vi "3D_Traverse_move_manual.vi"() -> ()   [LabVIEW 2020]
uses:
  Controls/Tunnel_Coordinates.ctl
  Trav_mode.ctl
  Controls/User_Specific_mode.ctl
  Globals/Constants_global.vi
panel:
  out "Current Traverse":string
  in  "Work in Tunnel Coordinates":T1
  in  "Traverse":u16(ring) items=["A_Tunnel", "A_Tunnel_Turntable", "Aero_Enclosure", "Aero_Pitch", "Aero_Sting", "Aero_ThroughWall", "Aero_Tunnel", "Angle_Calibrator", "B_Tunnel", "D_Tunnel", "dummy", "Dummy_Traverse", "EnFlo_Stack", "EnFlo_Trav1", "EnFlo_Trav3", "EnFlo_Trav4", "EnFlo_Tunnel", "EnFlo_Turntable", "F1_Wing_Angle", "Fast_Trav", "Fruit_Rig", "Laser_Disp_Scanner", "Laser_Meas_Traverse", "None", "Pitch_Traverse", "Pitch_Yaw", "PIV_Traverse", "Pressure_Port_1", "Pressure_Port_2", "Scanning Valve", "Soil_Rig", "Tank", "Trav_test"]
  in  "stop":bool
  in  "Increment":dbl=10.0
  in  "Z-":bool
  in  "Z+":bool
  in  "Y+":bool
  in  "Y-":bool
  in  "X+":bool
  in  "X-":bool
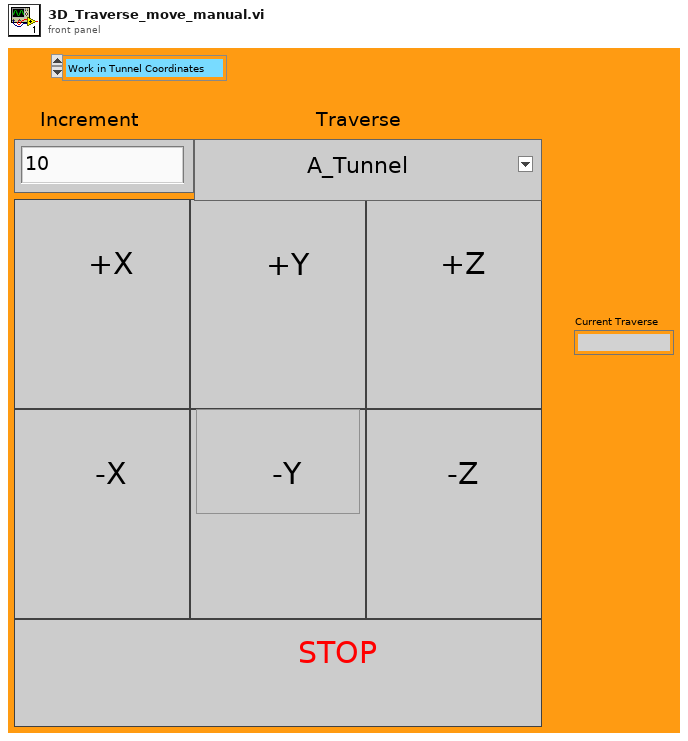
[diagram p1: front panel]
types:
  T1 = typedef "Tunnel_Coordinates.ctl" = enum16{"Work in Tunnel Coordinates", "Work in Model Coordinates"}
  T2 = typedef "User_Specific_mode.ctl" = enum16{"Check VI only", "Run VI"}
  T3 = typedef "Trav_mode.ctl" = enum16{"Move traverse", "Read traverse position", "Teach Position"}
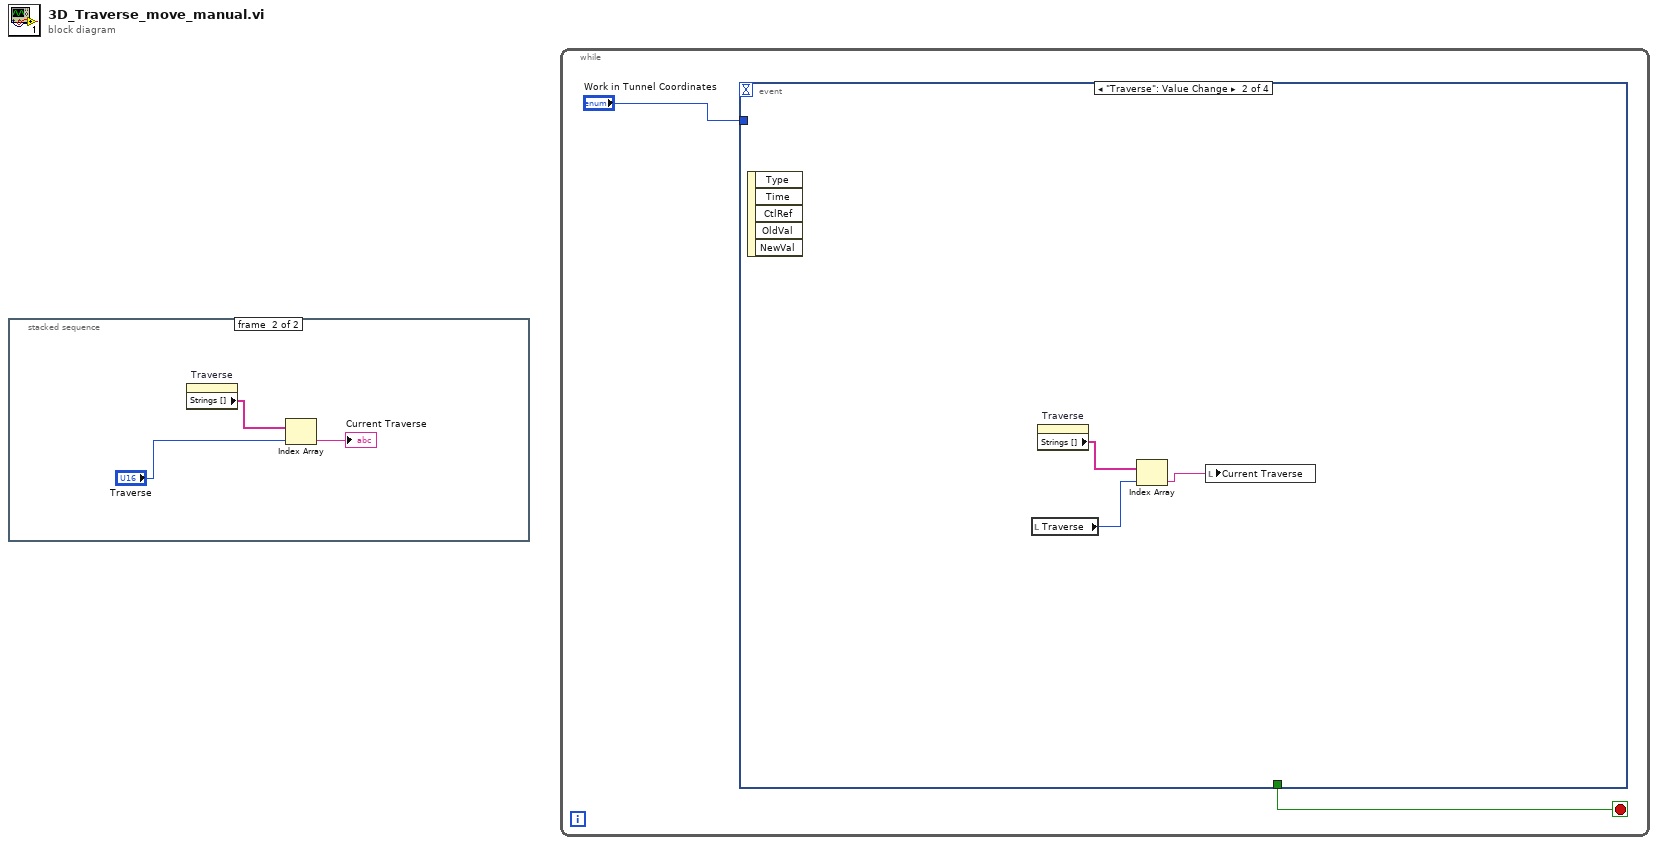
[diagram p0: block diagram]
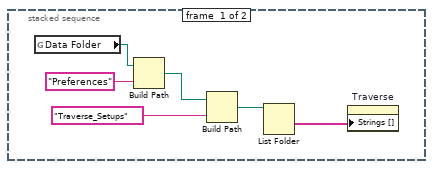
[diagram p2: hidden frame]
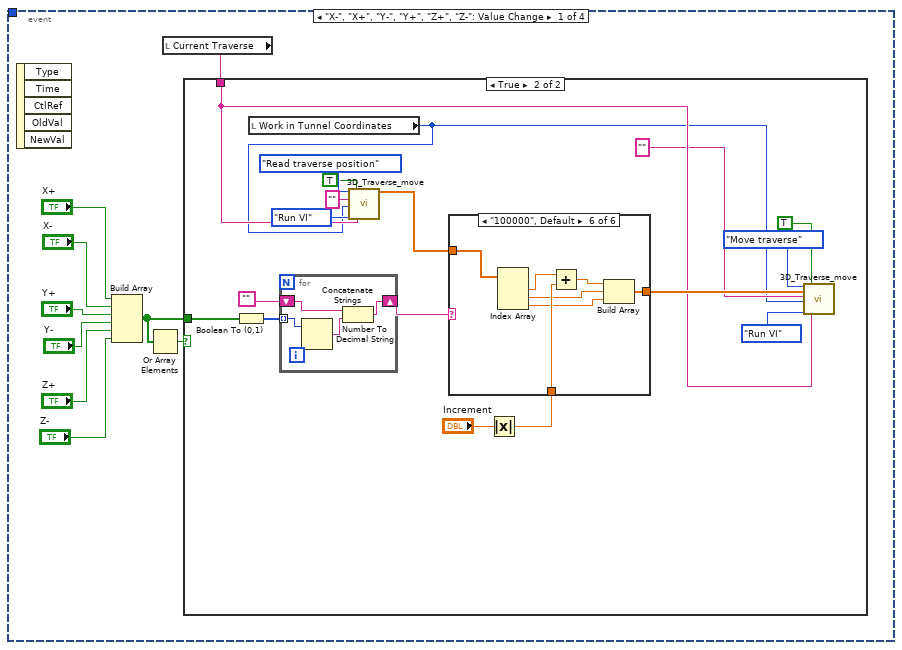
[diagram p3: hidden frame]
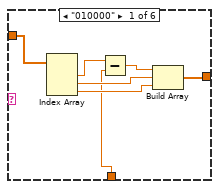
[diagram p5: hidden frame]
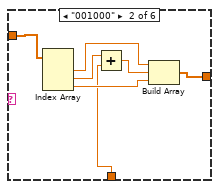
[diagram p6: hidden frame]
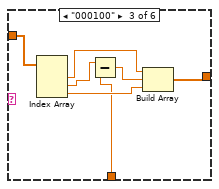
[diagram p7: hidden frame]
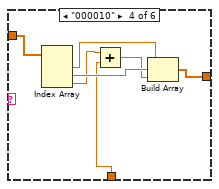
[diagram p8: hidden frame]
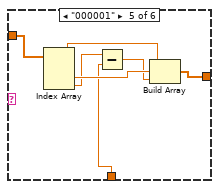
[diagram p9: hidden frame]
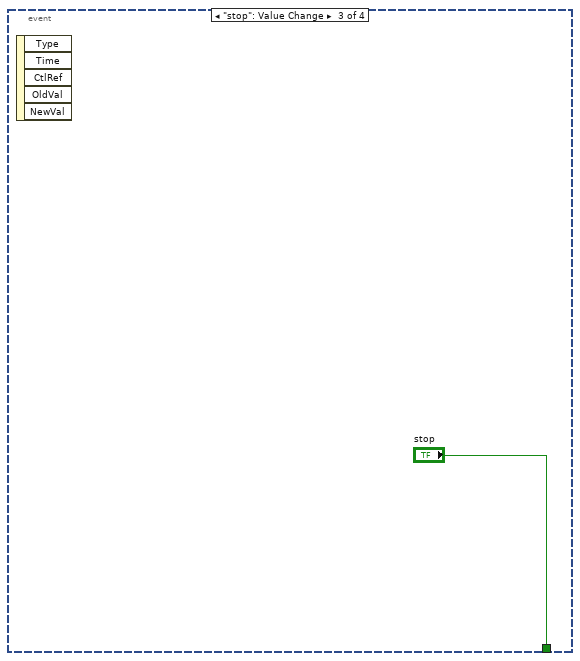
[diagram p10: hidden frame]
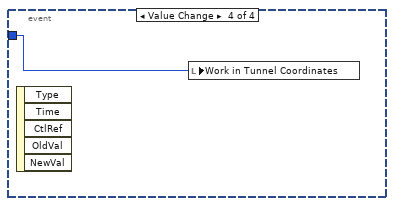
[diagram p11: hidden frame]
diagram:
  n1 = stacked-sequence {
    frame #0 {
      n2 = global read "Constants_global.vi" "Data Folder"() -> (w3:path)
      n3 = Build Path(base path=w3, name or relative path="Preferences") -> (appended path=w5:path)
      n4 = Build Path(base path=w5, name or relative path="Traverse_Setups") -> (appended path=w6:path)
      n5 = List Folder(path=w6) -> (folder names=w1:string[])  [unwired: 1 in, 5 out]
      n6 = property on="Traverse" class="Ring (strict)"("Strings []"=w1) -> ()  [unwired: 2 in, 2 out]
    }
    frame #1 {
      n7 = property on="Traverse" class="Ring (strict)"() -> ("Strings []"=w9:string[])  [unwired: 2 in, 2 out]
      n8 = Index Array(array=w9, index="Traverse") -> (element=→"Current Traverse":string)
    }
  }
  n9 = while {
    stop <- w11 stop-if-true
    n10 = event shown="[1] \"Traverse\": Value Change" {
      selector: _ -> [_ _ _ _]
      dyn-events: _ -> [_ _ _ _]
      timeout: _ -> [_ _ _ _]
      tunnel: [_ _ "stop" _] -> w11
      tunnel: "Work in Tunnel Coordinates" -> [_ _ _ w89]
      event "X-", "X+", "Y-", "Y+", "Z+", "Z-": Value Change {
        n11 = event-data() -> ()  [unwired: 1 in, 5 out]
        n12 = Build Array("X+", "X-", "Y+", "Y-", "Z+", "Z-") -> (w13:bool[])
        n13 = Or Array Elements(Boolean array=w13) -> (logical OR=w14:bool)
        n14 = local read "Current Traverse"() -> (w12:string)
        n15 = case shown="True" w14 {
          tunnel: w13 -> [_ w30]
          tunnel: w12 -> [_ w26]
          frame False {
          }
          frame True {
            n16 = Boolean To (0,1)(Boolean=w30) -> (0, 1=w37:i16[])
            n17 = local read "Work in Tunnel Coordinates"() -> (w21:T1)
            n18 = for {
              shift-right: [w41] -> w36
              shift-left: "" -> [w42]
              tunnel: w37 -> [w40] mode=indexing
              n19 = Number To Decimal String(number=w40) -> (decimal integer string=w39:string)  [unwired: 1 in]
              n20 = Concatenate Strings(w42, w39) -> (w41:string)
            }
            n21 = call "3D_Traverse_move.vi"("Mode"=Trav_mode."Read traverse position", "Extra command String"="", "Work in Tunnel Coordinates"=w21, "Simulate/Run"=User_Specific_mode."Run VI", "Route Checking?"=TRUE, "Traverse name"=w26) -> ("Trav Position achieved"=w27:sgl[])  [unwired: 10 in, 3 out]
            n22 = Absolute Value(x="Increment") -> (abs(x)=w34:dbl)
            n23 = case shown="\"100000\", Default" w36 {
              tunnel: w27 -> [w43 w55 w59 w69 w76 w84]
              tunnel: w34 -> [w44 w54 w58 w65 w75 w82]
              tunnel: [w45 w50 w57 w64 w71 w78] -> w33
              frame "010000" {
                n24 = Index Array(array=w43) -> (element #1=w49:sgl, element #2=w47:sgl, element #3=w46:sgl)  [unwired: 3 in]
                n25 = Subtract(x=w49, y=w44) -> (x-y=w48:dbl)
                n26 = Build Array(w48, w47, w46) -> (w45:dbl[])
              }
              frame "001000" {
                n27 = Index Array(array=w55) -> (element #1=w52:sgl, element #2=w51:sgl, element #3=w56:sgl)  [unwired: 3 in]
                n28 = Add(x=w51, y=w54) -> (x+y=w53:dbl)
                n29 = Build Array(w52, w53, w56) -> (w50:dbl[])
              }
              frame "000100" {
                n30 = Index Array(array=w59) -> (element #1=w60:sgl, element #2=w62:sgl, element #3=w63:sgl)  [unwired: 3 in]
                n31 = Subtract(x=w62, y=w58) -> (x-y=w61:dbl)
                n32 = Build Array(w60, w61, w63) -> (w57:dbl[])
              }
              frame "000010" {
                n33 = Index Array(array=w69) -> (element #1=w66:sgl, element #2=w70:sgl, element #3=w68:sgl)  [unwired: 3 in]
                n34 = Add(x=w68, y=w65) -> (x+y=w67:dbl)
                n35 = Build Array(w66, w70, w67) -> (w64:dbl[])
              }
              frame "000001" {
                n36 = Index Array(array=w76) -> (element #1=w72:sgl, element #2=w77:sgl, element #3=w74:sgl)  [unwired: 3 in]
                n37 = Subtract(x=w74, y=w75) -> (x-y=w73:dbl)
                n38 = Build Array(w72, w77, w73) -> (w71:dbl[])
              }
              frame "100000", Default {
                n39 = Index Array(array=w84) -> (element #1=w83:sgl, element #2=w80:sgl, element #3=w79:sgl)  [unwired: 3 in]
                n40 = Add(x=w83, y=w82) -> (x+y=w81:dbl)
                n41 = Build Array(w81, w80, w79) -> (w78:dbl[])
              }
            }
            n42 = call "3D_Traverse_move.vi"("Mode"=Trav_mode."Move traverse", "Position"=w33, "Extra command String"="", "Work in Tunnel Coordinates"=w21, "Simulate/Run"=User_Specific_mode."Run VI", "Route Checking?"=TRUE, "Traverse name"=w26) -> ()  [unwired: 9 in, 4 out]
          }
        }
      }
      event "Traverse": Value Change {
        n43 = event-data() -> ()  [unwired: 1 in, 5 out]
        n44 = local read "Traverse"() -> (w86:u16)
        n45 = property on="Traverse" class="Ring (strict)"() -> ("Strings []"=w87:string[])  [unwired: 2 in, 2 out]
        n46 = Index Array(array=w87, index=w86) -> (element=w85:string)
        n47 = local write "Current Traverse"(w85) -> ()
      }
      event "stop": Value Change {
        n48 = event-data() -> ()  [unwired: 1 in, 5 out]
      }
      event Value Change {
        n49 = event-data() -> ()  [unwired: 1 in, 5 out]
        n50 = local write "Work in Tunnel Coordinates"(w89) -> ()
      }
    }
  }
